vi "CAL-Probe Tube Cal Path.vi"(5 "Probe Tube Folder":path=path "C:/Data/Probe Tube Calibrations", 7 "Acoustic System":string, 11 "error in (no error)":errorcluster) -> (6 "Probe Tube Cal Path":path, 15 "error out":errorcluster)   [LabVIEW 2020]
uses:
  SubVIs/Calibration Globals.vi
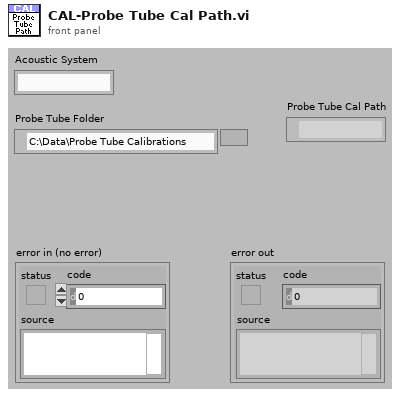
[diagram p1: front panel]
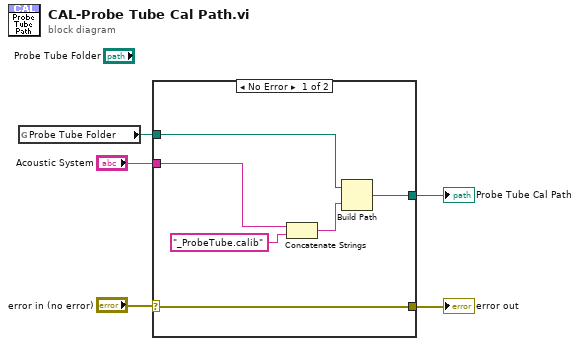
[diagram p0: block diagram]
diagram:
  n1 = global read "Calibration Globals.vi" "Probe Tube Folder"() -> (w1:path)
  n2 = case shown="No Error" "error in (no error)" {
    selector: "error in (no error)" -> [w7 w12]
    tunnel: "Acoustic System" -> [w6 _]
    tunnel: w1 -> [w10 _]
    tunnel: [w8 _] -> w3
    tunnel: [w7 w12] -> w2
    frame No Error {
      n3 = Concatenate Strings(w6, "_ProbeTube.calib" ("string")) -> (w9:string)
      n4 = Build Path(base path=w10, name or relative path=w9) -> (appended path=w8:path)
    }
    frame Error {
    }
  }
  "error out" <- w2
  "Probe Tube Cal Path" <- w3
